vi "Tag Metadata Check New.vi"(0 "Tags":string[](array[string]), 5 "Sorted Tags":string[](array[string]), 7 "First Letters":string[](array[string]), 9 "Letter Indicies":i32[](array[numeric])) -> (8 "New Tags":string[](array[string]), 15 "New Tags Bool":bool)   [LabVIEW 2020]
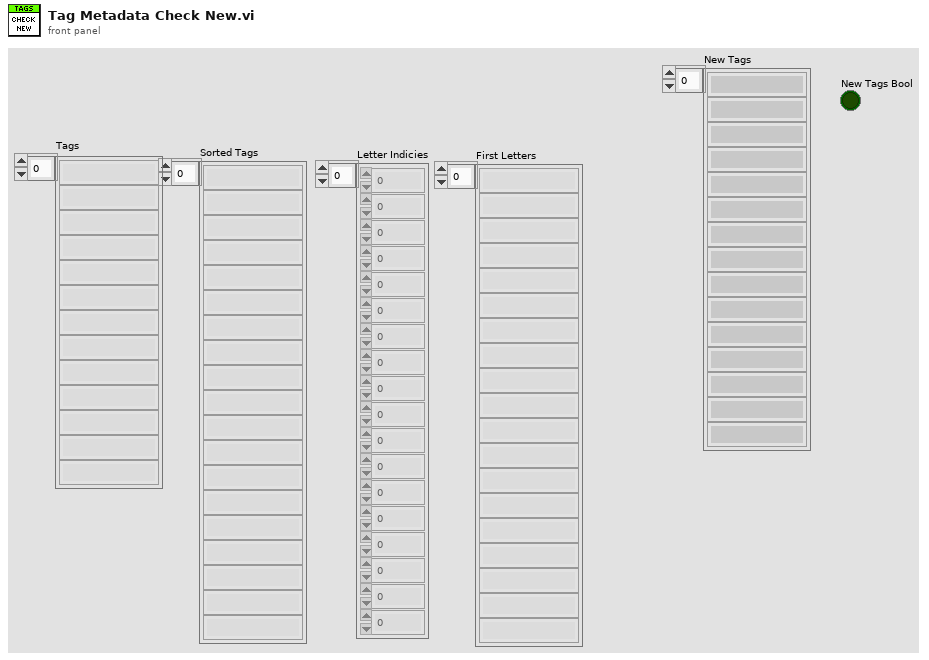
[diagram p1: front panel]
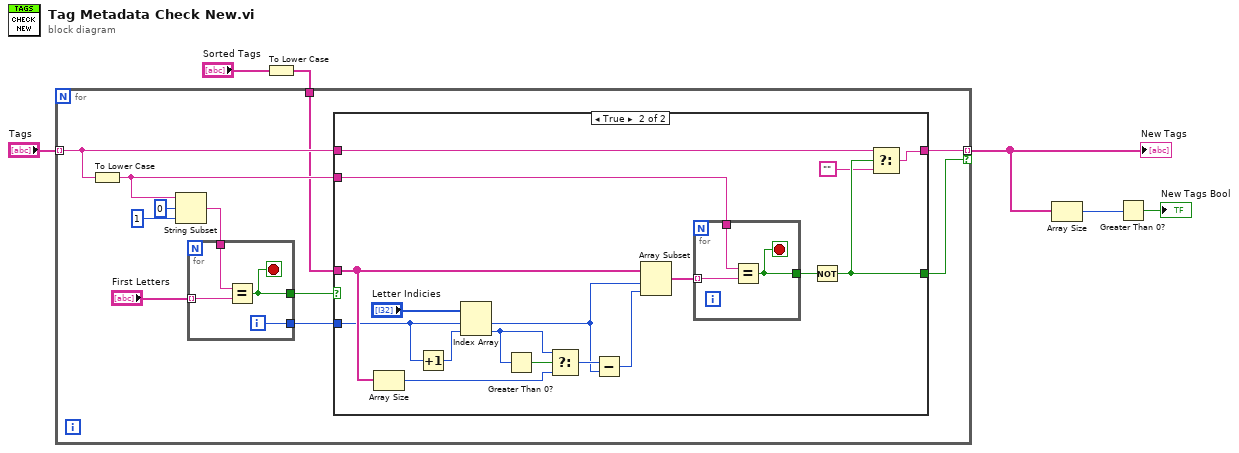
[diagram p0: block diagram]
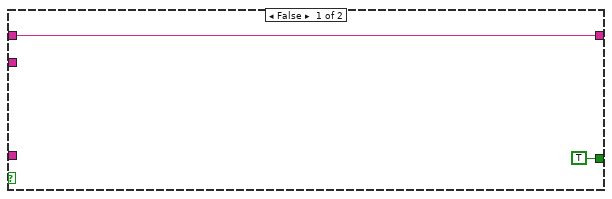
[diagram p2: hidden frame]
diagram:
  n1 = To Lower Case(string="Sorted Tags") -> (all lower case string=w4:string[])
  n2 = for {
    tunnel: "Tags" -> [w10] mode=indexing
    tunnel: [w9] -> w3 mode=indexing if=w8
    tunnel: w4 -> [w7]
    n3 = To Lower Case(string=w10) -> (all lower case string=w11:string)
    n4 = String Subset(string=w11, offset (0)=0, length (rest)=1 ("length (rest)")) -> (substring=w14:string)
    n5 = for {
      tunnel: "First Letters" -> [w43] mode=indexing
      tunnel: w14 -> [w42]
      tunnel: [w41] -> w13
      tunnel: [w40] -> w12
      i -> [w40]
      stop <- w41 stop-if-true
      n6 = Equal?(x=w42, y=w43) -> (x = y?=w41:bool)
    }
    n7 = case shown="True" w13 {
      tunnel: w7 -> [_ w30]
      tunnel: w12 -> [_ w27]
      tunnel: w10 -> [w19 w22]
      tunnel: [w19 w21] -> w9
      tunnel: w11 -> [_ w25]
      tunnel: [TRUE w23] -> w8
      frame False {
      }
      frame True {
        n8 = Array Size(array=w30) -> (size(s)=w32:i32)
        n9 = Increment(x=w27) -> (x+1=w35:i32)
        n10 = Index Array(array="Letter Indicies", index #1=w27, index #2=w35) -> (element #1=w28:i32, element #2=w33:i32)
        n11 = Greater Than 0?(x=w33) -> (x > 0?=w34:bool)
        n12 = Select(t=w33, s=w34, f=w32) -> (s? t:f=w31:i32)
        n13 = Subtract(x=w31, y=w28) -> (x-y=w29:i32)
        n14 = Array Subset(array=w30, index=w28, length=w29) -> (w26:string[])
        n15 = for {
          tunnel: w26 -> [w39] mode=indexing
          tunnel: w25 -> [w38]
          tunnel: [w37] -> w24
          stop <- w37 stop-if-true
          n16 = Equal?(x=w38, y=w39) -> (x = y?=w37:bool)
        }
        n17 = Not(x=w24) -> (.not. x?=w23:bool)
        n18 = Select(t=w22, s=w23, f="") -> (s? t:f=w21:string)
      }
    }
  }
  "New Tags" <- w3
  n19 = Array Size(array=w3) -> (size(s)=w2:i32)
  n20 = Greater Than 0?(x=w2) -> (x > 0?=→"New Tags Bool":bool)
